vi "poly_linspace_DBL.vi"(6 "inclusive? (T)":bool=TRUE, 8 "xN":dbl, 9 "N":i32, 10 "x0":dbl) -> (1 "linspace out":dbl[](array[numeric]))   [LabVIEW 2015]
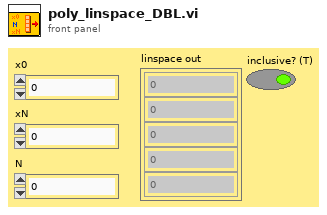
[diagram p1: front panel]
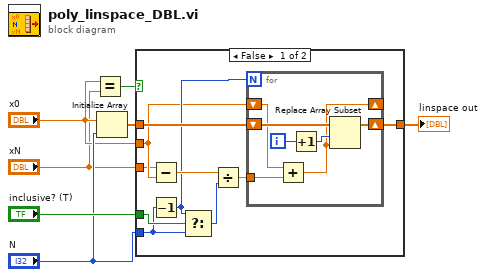
[diagram p0: block diagram]
diagram:
  n1 = Equal?(x="x0", y="xN") -> (x = y?=w1:bool)
  n2 = Initialize Array("x0", "N") -> (w7:dbl[])
  n3 = case shown="False" w1 {
    tunnel: w7 -> [w17 w25]
    tunnel: [w16 w25] -> w6
    tunnel: "inclusive? (T)" -> [w14 _]
    tunnel: "N" -> [w10 _]
    tunnel: "x0" -> [w9 _]
    tunnel: "xN" -> [w8 _]
    frame False {
      n4 = Subtract(x=w8, y=w9) -> (x-y=w12:dbl)
      n5 = Decrement(x=w10) -> (x-1=w11:i32)
      n6 = Select(t=w11, s=w14, f=w10) -> (s? t:f=w13:i32)
      n7 = Divide(x=w12, y=w13) -> (x/y=w15:dbl)
      n8 = for {
        N: w11 -> [_]
        shift-right: [w21] -> w16
        shift-left: w17 -> [w24]
        shift-right: [w18] -> _
        shift-left: w9 -> [w23]
        tunnel: w15 -> [w22]
        i -> [w20]
        n9 = Add(x=w23, y=w22) -> (x+y=w18:dbl)
        n10 = Increment(x=w20) -> (x+1=w19:i32)
        n11 = Replace Array Subset(array=w24, new element=w18, index=w19) -> (w21:dbl[])
      }
    }
    frame True {
    }
  }
  "linspace out" <- w6
